vi "Write Channel Array.vi"(8 "error in (no error)":errorcluster, 10 "Channel Array":refnum<class "CIFChannels.lvclass">[](array[class]), 11 "CIFCorePlugin in":refnum<class "CIFCorePlugin.lvclass">) -> (0 "error out":errorcluster, 3 "CIFCorePlugin out":refnum<class "CIFCorePlugin.lvclass">)   [LabVIEW 2021, in "CIFCorePlugin.lvclass"]
uses:
  CIFCorePlugin.lvclass
  CIFCorePlugin.lvclass/CIFCorePlugin.ctl
  Channels/CIFChannelMng/CIFChannelMng.lvclass
  <vilib>/CIF Foundation/CIF Channels Core/CIFChannels/CIFChannels.lvclass
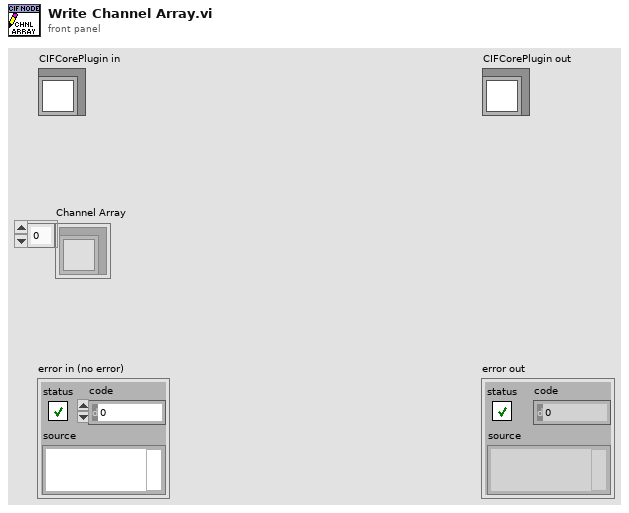
[diagram p1: front panel]
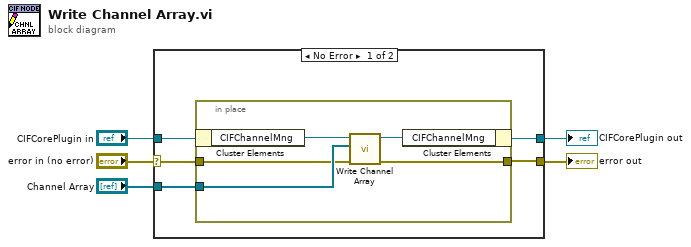
[diagram p0: block diagram]
diagram:
  n1 = case shown="No Error" "error in (no error)" {
    selector: "error in (no error)" -> [w7 w16]
    tunnel: [w6 w16] -> w4
    tunnel: [w8 w17] -> w2
    tunnel: "CIFCorePlugin in" -> [w9 w17]
    tunnel: "Channel Array" -> [w10 _]
    frame No Error {
      n2 = in-place {
        in-place-border: w10 -> [w15]
        in-place-border: w7 -> [w12]
        in-place-border: [w11] -> w6
        n3 = in-place-cluster #1(w9) -> ("CIFChannelMng"=w14:refnum<class "CIFChannelMng.lvclass">)
        n4 = call "Write Channel Array.vi"("error in (no error)"=w12, "Channel Array"=w15, "CIFChannelMng in"=w14) -> ("error out"=w11:errorcluster, "CIFChannelMng out"=w13:refnum<class "CIFChannelMng.lvclass">)  [unwired: 7 in]
        n5 = in-place-cluster #1("CIFChannelMng"=w13) -> (w8:refnum<class "CIFCorePlugin.lvclass">)
      }
    }
    frame Error {
    }
  }
  "error out" <- w4
  "CIFCorePlugin out" <- w2
